vi "AUTOFOCUS_calculate_derivative.vi"(4 "z":dbl, 5 "Dimension size":i32, 6 "error in":errorcluster, 7 "iteration":i32, 8 "X":dbl[](array[numeric]), 9 "Y":dbl[](array[numeric])) -> (0 "error out":errorcluster, 1 "dx/dt":dbl format="%0.2f", 2 "Y out":dbl[](array[numeric]), 3 "iteration out":i32)   [LabVIEW 2015]
uses:
  <vilib>/Analysis/6fits.llb/Curve Fitting Criteria.ctl
  <vilib>/Analysis/NI_AALPro.lvlib
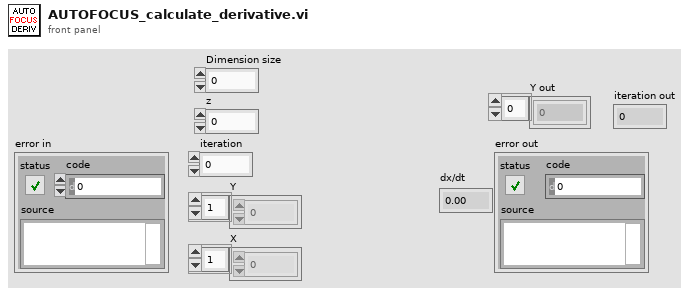
[diagram p1: front panel]
types:
  T1 = typedef "NI_AALPro.lvlib/Curve Fitting Criteria.ctl" = u16
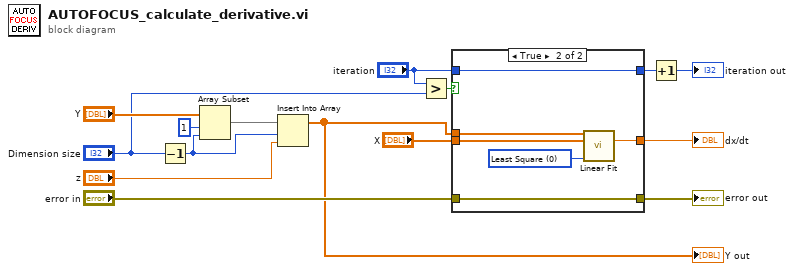
[diagram p0: block diagram]
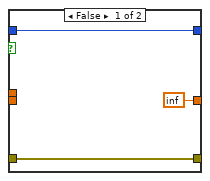
[diagram p2: hidden frame]
diagram:
  n1 = Decrement(x="Dimension size") -> (x-1=w7:i32)
  n2 = Array Subset(array="Y", index=1, length=w7) -> (w8:dbl[])
  n3 = Insert Into Array(array=w8, index=w7, new element="z") -> (w5:dbl[])
  "Y out" <- w5
  n4 = Greater?(x="iteration", y="Dimension size") -> (0:w15:bool)
  n5 = case shown="True" w15 {
    tunnel: w5 -> [_ w23]
    tunnel: "X" -> [_ w22]
    tunnel: [inf w21] -> w13
    tunnel: "error in" -> [w17 w20]
    tunnel: [w17 w20] -> w11
    tunnel: "iteration" -> [w16 w19]
    tunnel: [w16 w19] -> w2
    frame False {
    }
    frame True {
      w24 = T1 0 items=["Least Square", "Least Absolute Residual", "Bisquare"] ("method")
      n6 = call <vilib>:"Linear Fit.vi"("Y"=w23, "X"=w22, "method"=w24) -> ("slope"=w21:dbl)  [unwired: 8 in, 4 out]
    }
  }
  "dx/dt" <- w13
  "error out" <- w11
  n7 = Increment(x=w2) -> (x+1=→"iteration out":i32)
